vi "Write MTi Theta Offset.vi"(8 "error in (no error)":errorcluster, 10 "MTi Theta Offset":dbl[](array[numeric])=[0.0, 0.0, 0.0], 11 "Attitude Observer in":refnum<class "Attitude Observer.lvclass">) -> (0 "error out":errorcluster, 3 "Attitude Observer out":refnum<class "Attitude Observer.lvclass">)   [LabVIEW 2014, in "Observer Library.lvlib" / "Attitude Observer.lvclass"]
uses:
  Attitude Observer.lvclass
  Attitude Observer.lvclass/Attitude Observer.ctl
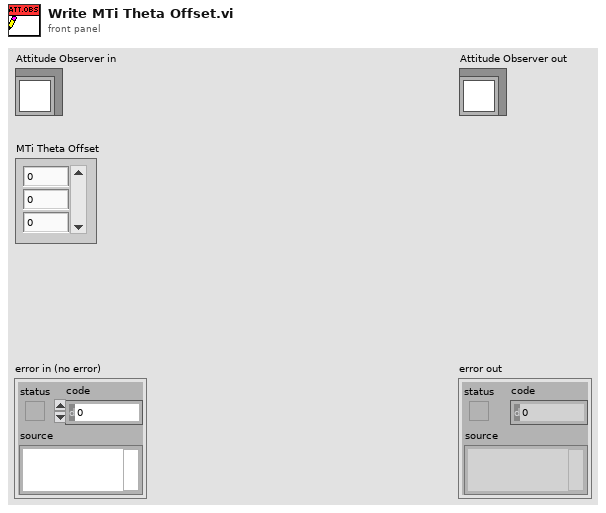
[diagram p1: front panel]
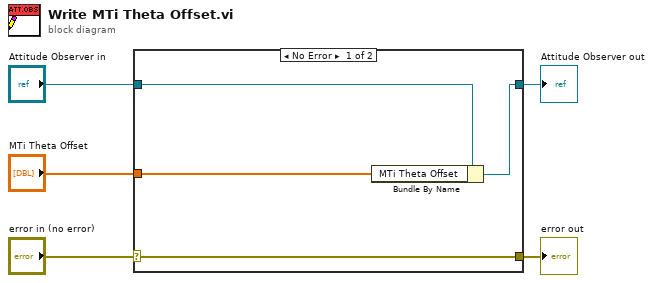
[diagram p0: block diagram]
diagram:
  n1 = case shown="No Error" "error in (no error)" {
    selector: "error in (no error)" -> [w9 w10]
    tunnel: [w9 w10] -> w4
    tunnel: [w7 w11] -> w2
    tunnel: "Attitude Observer in" -> [w8 w11]
    tunnel: "MTi Theta Offset" -> [w6 _]
    frame No Error {
      n2 = Bundle By Name(cluster=w8, "MTi Theta Offset"=w6) -> (w7:refnum<class "Attitude Observer.lvclass">)
    }
    frame Error {
    }
  }
  "error out" <- w4
  "Attitude Observer out" <- w2
